vi "Fire User Event - Error.vi"(8 "error in (no error)":errorcluster, 10 "Error Type":T1, 11 "UE Error":refnum<user-event>) -> (0 "error out":errorcluster)   [LabVIEW 2017, in "User Events.lvlib"]
doc: "Send the Error event to the Event Handling Loop"
uses:
  User Events.lvlib
  Error Handler/Controls/Error EventData.ctl
  Error Handler/Controls/Error Type.ctl
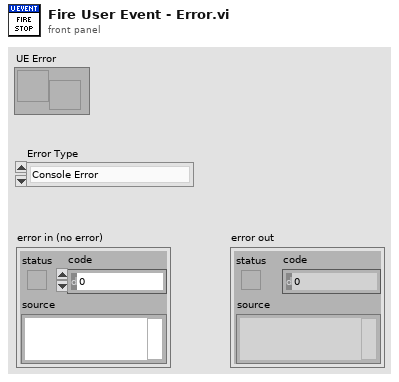
[diagram p1: front panel]
types:
  T1 = typedef "Error Type.ctl" = enum16{"Console Error", "Sensor Interface IO Error", "Process Step Error"}
  T2 = typedef "Error EventData.ctl" = cluster{"Error Type":T1, "error in (no error)":errorcluster}
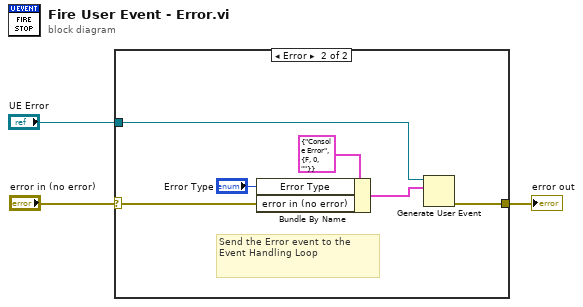
[diagram p0: block diagram]
diagram:
  n1 = case shown="Error" "error in (no error)" {
    selector: "error in (no error)" -> [w4 w5]
    tunnel: [w4 w10] -> w3
    tunnel: "UE Error" -> [_ w9]
    frame No Error {
    }
    frame Error {
      # "Send the Error event to the Event Handling Loop"
      n2 = Bundle By Name(cluster=T2 {"Error Type"=enum."Console Error", "error in (no error)"={"status"=FALSE, "code"=0, "source"=""}} ("Error Event Data"), "Error Type"="Error Type", "error in (no error)"=w5) -> (w7:T2)
      n3 = Generate User Event(user event=w9, event data cluster=w7) -> (error out=w10:errorcluster)  [unwired: 2 in, 1 out]
    }
  }
  "error out" <- w3
